vi "Example.vi"() -> ()   [LabVIEW 2019, in "Stand.lvclass"]
uses:
  Stand.lvclass
  ConfigJSON_class/ConfigJSON.lvclass
  MessageAMC_class/MessageAMC.lvclass
  <vilib>/NI/AMC/AMC.lvlib
  Logger_class/Logger.lvclass
  Proccess_class/Proccess.lvclass
  TypeDef/State.ctl
  Shared Data.ctl
  D:/GIT H4000/H4000/src/ConfigInterface_class/ConfigInterface.lvclass
  D:/GIT H4000/H4000/src/MessageInterface_class/MessageInterface.lvclass
  D:/GIT H4000/H4000/src/Device_class/Device.lvclass
  D:/GIT H4000/H4000/src/Proccess_class/Proccess.lvclass
  SharedData DVR.ctl
panel:
  out "SharedData DVR":T1
  in  "stop":bool
  out "error out":errorcluster
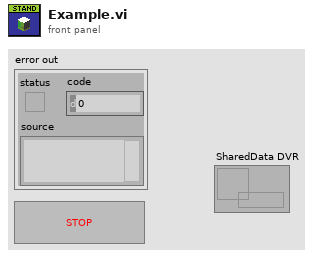
[diagram p1: front panel]
types:
  T1 = typedef "Stand.lvclass/SharedData DVR.ctl" = refnum<data-value>
  T2 = typedef "Stand.lvclass/Shared Data.ctl" = cluster{"State":T3}
  T3 = typedef "State.ctl" = enum16{"INIT", "IDLE", "CHANNEL_TESTING", "OIL_FILLING", "PREPARE_TO_HI_PRESS", "HI_PRESSURE", "ALARM", "HI PRESSURE TEST"}
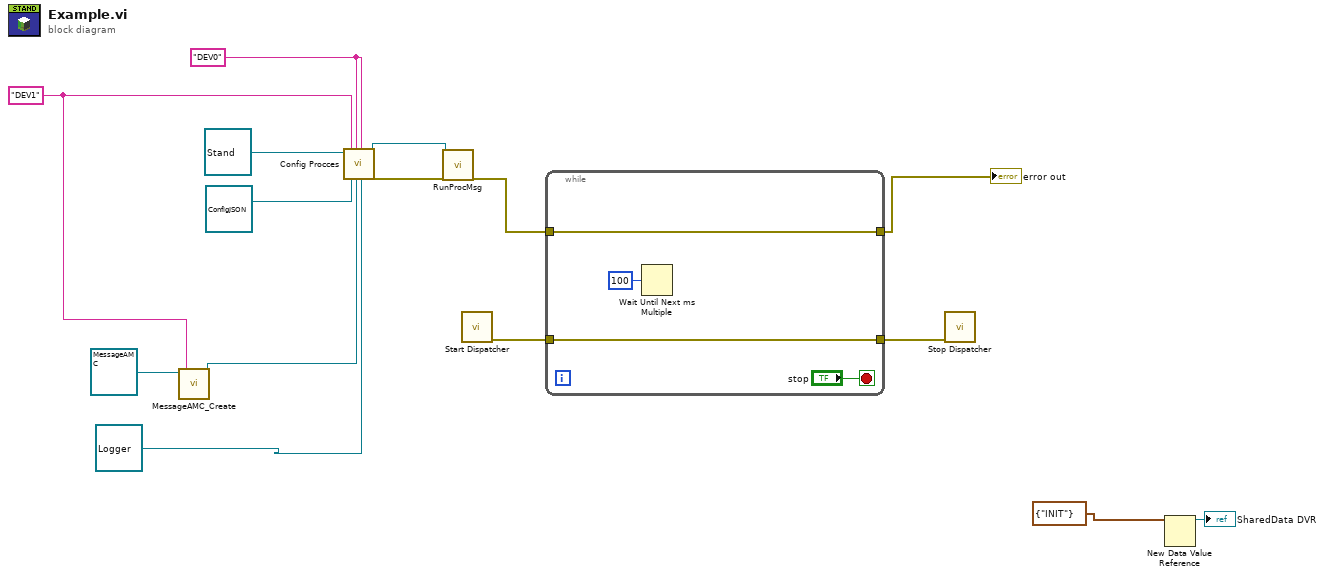
[diagram p0: block diagram]
diagram:
  w3 = "DEV0" ("ParentName")
  w4 = "DEV1" ("Name")
  n1 = call "MessageAMC_Create.vi"("reference in"=refnum<class "MessageAMC.lvclass"> refnum ("MessageAMC"), "message queue name"=w4) -> ("amc"=w6:refnum<class "MessageAMC.lvclass">)  [unwired: 16 in, 1 out]
  n2 = call "Config Procces.vi"("reference in"=refnum<class "Stand.lvclass"> refnum, "Name"=w4, 7:refnum<class "ConfigJSON.lvclass"> refnum ("ConfigJSON"), "ParentName"=w3, 9:w6, "Description"=w3, "Logger"=refnum<class "Logger.lvclass"> refnum) -> ("reference out"=w9:refnum<class "Stand.lvclass">, "error out"=w8:errorcluster)  [unwired: 11 in]
  n3 = call-dynamic "RunProcMsg.vi"("reference in"=w9, "error in (no error)"=w8) -> ("error out"=w14:errorcluster)  [unwired: 16 in, 1 out]
  n4 = call <vilib>:"Start Dispatcher.vi"() -> ("error out"=w11:errorcluster)  [unwired: 13 in, 2 out]
  n5 = while {
    tunnel: w14 -> [w19]
    tunnel: [w19] -> w13
    tunnel: [w16] -> w12
    tunnel: w11 -> [w16]
    stop <- "stop" stop-if-true
    n6 = Wait Until Next ms Multiple(millisecond multiple=u32 100) -> ()  [unwired: 1 out]
  }
  "error out" <- w13
  n7 = call <vilib>:"Stop Dispatcher.vi"("error in"=w12) -> ()  [unwired: 14 in, 1 out]
  n8 = New Data Value Reference(data value=T2 {"State"=enum."INIT"} ("Shared Data")) -> (data value reference=→"SharedData DVR":refnum<data-value>)  [unwired: 1 in, 1 out]
